vi "Method_Const.vi"(4 "Value":sgl, 5 "Input A":refnum<class "Abs_Single Float.lvclass">) -> (1 "Result":T1)   [LabVIEW 2021, in "Subtract_SGL.lvclass"]
uses:
  Subtract_SGL.lvclass
  Abs_Types/Single Float/Abs_Single Float.lvclass
  C:/Program Files (x86)/National Instruments/LabVIEW 2021/vi.lib/TSA/Abstract Data Classes/Abs_Types/Numeric/Abs_Numeric.lvclass
  Abs Type.ctl
  C:/TSA/LV_Abstract/Source/Functions/Support/Function/Two Terminal/SGL/AbsFunc_Two Term_SGL.lvclass
  C:/Program Files (x86)/National Instruments/LabVIEW 2021/vi.lib/TSA/Abstract Data Classes/Abs_Types/Single Float/Abs_Single Float.lvclass
  Support/Function/Two Terminal/SGL/AbsFunc_Two Term_SGL.lvclass/AbsFunc_Two Term_SGL.ctl
  Support/Function/Two Terminal/SGL/Properties/Write Numeric A.vi
  Support/Function/Two Terminal/SGL/Properties/Write Numeric B.vi
  Constants/Support/SGL/Const_SGL.lvclass
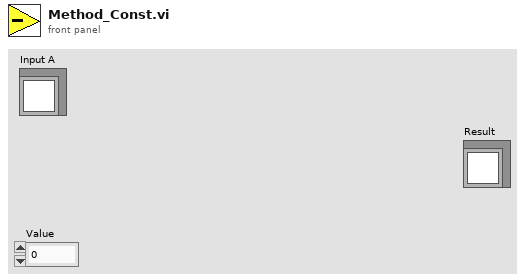
[diagram p1: front panel]
types:
  T1 = typedef "Subtract_SGL.lvclass/Abs Type.ctl" = refnum<class "Abs_Single Float.lvclass">
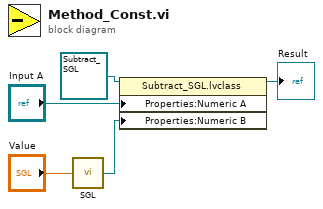
[diagram p0: block diagram]
diagram:
  n1 = call "SGL.vi"("Value"="Value") -> ("Constant"=w2:refnum<class "Abs_Single Float.lvclass">)  [unwired: 4 in]
  n2 = property class="Subtract_SGL.lvclass"(reference=refnum<class "Subtract_SGL.lvclass"> refnum ("Subtract_DBL.lvclass"), "Properties:Numeric A"="Input A", "Properties:Numeric B"=w2) -> (reference out=→"Result":refnum<class "Subtract_SGL.lvclass">)  [unwired: 1 in, 1 out]
